vi "5_Creating_complex_analog_and_digital_sequences.vi"() -> ()   [LabVIEW 2014]
uses:
  <vilib>/Swabian Instruments/Pulse Streamer/PulseStreamer/PulseStreamer/typedefs/typedef_TriggerStart.ctl
  <vilib>/Swabian Instruments/Pulse Streamer/PulseStreamer/PulsePattern/PulsePattern.lvclass
  <vilib>/Swabian Instruments/Pulse Streamer/PulseStreamer/AnalogPattern/AnalogPattern.lvclass
  <vilib>/Swabian Instruments/Pulse Streamer/PulseStreamer/typedefs/typedef_ChannelNumber.ctl
  <vilib>/Swabian Instruments/Pulse Streamer/PulseStreamer/typedefs/typedef_OutputState.ctl
  <vilib>/Swabian Instruments/Pulse Streamer/PulseStreamer/Sequence/Sequence.lvclass/Sequence.ctl
  <vilib>/Swabian Instruments/Pulse Streamer/PulseStreamer/Pattern/Read total duration.vi
  <vilib>/Swabian Instruments/Pulse Streamer/PulseStreamer/PulseStreamer/stream/stream (Sequence).vi
  <vilib>/Swabian Instruments/Pulse Streamer/PulseStreamer/PulseStreamer/PulseStreamer.lvclass
  <vilib>/Swabian Instruments/Pulse Streamer/PulseStreamer/Sequence/Sequence.lvclass
  <vilib>/Swabian Instruments/Pulse Streamer/PulseStreamer/PulseStreamer.lvlib
panel:
  in  "ip":string="pulsestreamer"
  out "Total Duration [ns]":i64
  in  "Digital Pattern\nDuration [ns] & Level":cluster{"Duration [ns]":u64, "State":bool}[](array[cluster])=[{"Duration [ns]"=1000, "State"=FALSE}, {"Duration [ns]"=500, "State"=TRUE}, {"Duration [ns]"=200, "State"=FALSE}, {"Duration [ns]"=300, "State"=TRUE}, {"Duration [ns]"=100, "State"=FALSE}]
  in  "Level 3":bool
  in  "Duration 3":i64=250
  out "error out":errorcluster
  in  "nRuns":i64=1000
  in  "Start Trigger":T1
  in  "Repeat sequence":u32=5
  in  "Voltage A ch0-2":dbl min=-1.0 max=1.0
  in  "Voltage A ch0-1":dbl=1.0 min=-1.0 max=1.0
  in  "Duration A ch0-2":i64
  in  "Duration A ch0-1":i64=100
  in  "Duration 2":i64=500
  in  "Duration 1":i64=1000
  in  "Level 2":bool=TRUE
  in  "Level 1":bool
  # "This example demonstrates how to program each channel individually and how to combine them into sequence. \nThe durations of each pulse are automatically split so that the Generated sequence has the Run Length Encoding (RLE).\nThe total duration of a sequence has the length of the longest duration of all channels. \nThis example also shows few powerful techniques on how prepared sequences can be combined and repeated."
  # "INPUT SECTION"
  # "RESULT SECTION"
  # "Level 1"
  # "Level 2"
  # "Level 3"
  # "Duration"
  # "The longest duration is from channel 'Digital 0' and hence,\n this channel determines the total duration."
  # "either add single pulses"
  # "Digital 0"
  # "or a array of cluster\ntop: duration\nbutton: state [1: high, 0: low]"
  # "Digital 1"
  # "Level 1"
  # "Level 2"
  # "The very same is possible for the analog channels. Here only the method to add single pulses is shown.\nRemark:\nAdding a Pulse of duration 0 might be useful because this state will be padded until the maximum duration of all channels is reached."
  # "Duration"
  # "Analog 0"
  # "Sequence class has a repeat method which duplicates sequence data."
  # "StartTrigger: IMMEDIATE - starts streaming immediately after data received\nSOFTWARE - use \"startNow.vi\" as software trigger\nHW_RAISING, HW_FALLING, HW_RISING_AND_FALLING - tell Pulse Streamer to trigger by signal connected to \"Trigger\" input"
  # "If there is only one sequence 'nRuns' from the 'stream' method should\nbe always used, because with 'Repeat' the data transferred to the \nPulsestreamer is repeated 'Repeat' times whereas nRuns sends the sequence\nonly once.\nRepeat >1 should be used when several sequences are combined and \neach sequence needs to be repeated."
  # "Here you can define the state to set after the sequence\n streaming has finished."
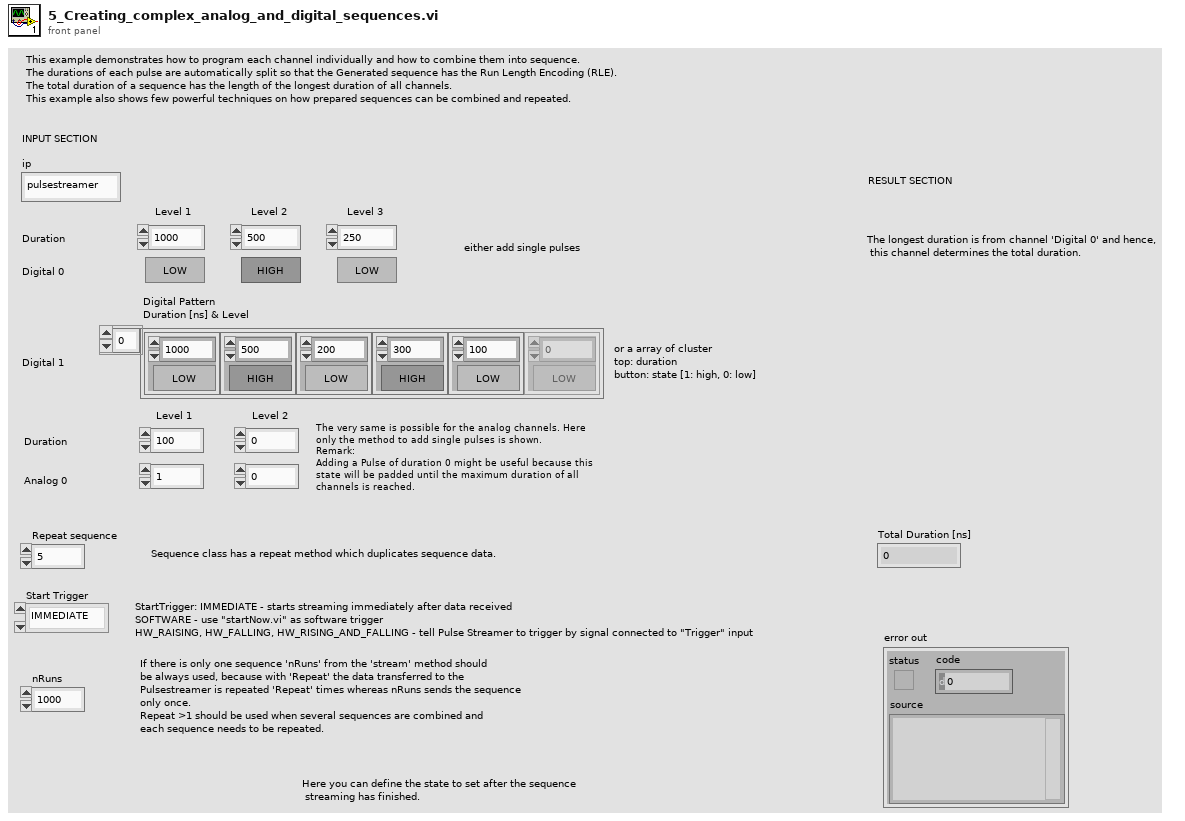
[diagram p1: front panel]
types:
  T1 = typedef "PulseStreamer.lvlib/PulseStreamer.lvclass/typedef_TriggerStart.ctl" = enum16{"IMMEDIATE", "SOFTWARE", "HW_RISING", "HW_FALLING", "HW_RISING_AND_FALLING"}
  T2 = typedef "PulseStreamer.lvlib/typedef_OutputState.ctl" = cluster{"channels":T3[], "a0":dbl, "a1":dbl}
  T3 = typedef "PulseStreamer.lvlib/typedef_ChannelNumber.ctl" = i16
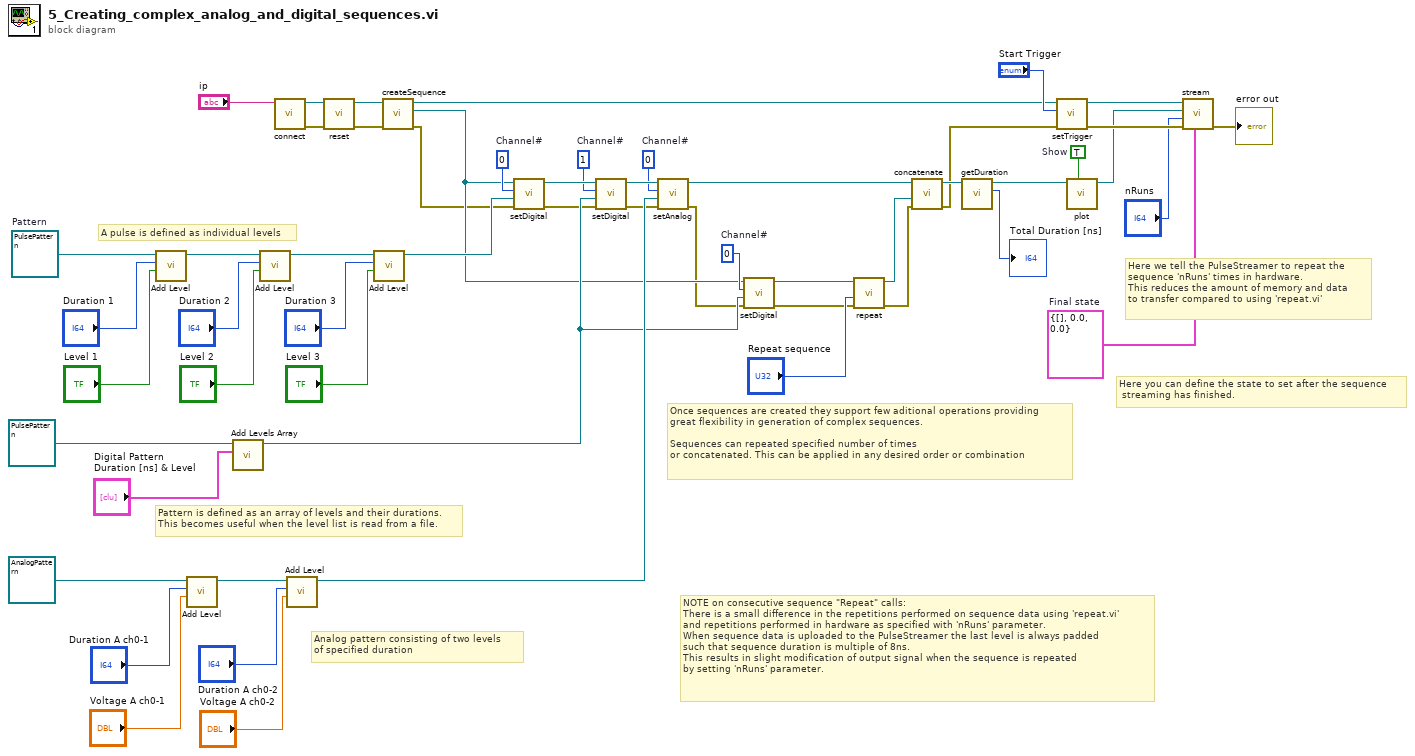
[diagram p0: block diagram]
diagram:
  w21 = T2 {"channels"=[], "a0"=0.0, "a1"=0.0}  # Final state
  w14 = TRUE  # Show
  w27 = T3 0  # Channel#
  w29 = T3 0  # Channel#
  w30 = T3 1  # Channel#
  w32 = T3 0  # Channel#
  w48 = refnum<class "PulsePattern.lvclass"> refnum  # Pattern
  # "Here you can define the state to set after the sequence\n streaming has finished."
  # "A pulse is defined as individual levels"
  # "NOTE on consecutive sequence \"Repeat\" calls: \nThere is a small difference in the repetitions performed on sequence data using 'repeat.vi'\nand repetitions performed in hardware as specified with 'nRuns' parameter.\nWhen sequence data is uploaded to the PulseStreamer the last level is always padded \nsuch that sequence duration is multiple of 8ns. \nThis results in slight modification of output signal when the sequence is repeated \nby setting 'nRuns' parameter."
  # "Here we tell the PulseStreamer to repeat the \nsequence 'nRuns' times in hardware.\nThis reduces the amount of memory and data\nto transfer compared to using 'repeat.vi'"
  # "Analog pattern consisting of two levels \nof specified duration"
  # "Pattern is defined as an array of levels and their durations.\nThis becomes useful when the level list is read from a file."
  # "Once sequences are created they support few aditional operations providing\ngreat flexibility in generation of complex sequences.\n\nSequences can repeated specified number of times \nor concatenated. This can be applied in any desired order or combination"
  n1 = call <vilib>:"Add Level.vi"("Level"="Level 1", "Duration"="Duration 1", "Digital Sequence in"=w48) -> ("Digital Sequence out"=w55:refnum<class "PulsePattern.lvclass">)  [unwired: 8 in]
  n2 = call <vilib>:"Add Level.vi"("Voltage"="Voltage A ch0-1", "Duration"="Duration A ch0-1", "Analog Sequence in"=refnum<class "AnalogPattern.lvclass"> refnum ("Analog Sequence.lvclass")) -> ("Analog Sequence out"=w53:refnum<class "AnalogPattern.lvclass">)  [unwired: 8 in]
  n3 = call-dynamic "Add Levels Array.vi"("Array of (Duration [ns], Level [T/F])"="Digital Pattern\nDuration [ns] & Level", "Digital Sequence in"=refnum<class "PulsePattern.lvclass"> refnum ("Digital Sequence.lvclass")) -> ("Digital Sequence out"=w25:refnum<class "PulsePattern.lvclass">)  [unwired: 9 in]
  n4 = call <vilib>:"Add Level.vi"("Level"="Level 2", "Duration"="Duration 2", "Digital Sequence in"=w55) -> ("Digital Sequence out"=w49:refnum<class "PulsePattern.lvclass">)  [unwired: 8 in]
  n5 = call <vilib>:"connect.vi"("ip"="ip") -> ("error out"=w23:errorcluster, "Pulse Streamer out"=w24:refnum<class "PulseStreamer.lvclass">)  [unwired: 9 in]
  n6 = call <vilib>:"Add Level.vi"("Voltage"="Voltage A ch0-2", "Duration"="Duration A ch0-2", "Analog Sequence in"=w53) -> ("Analog Sequence out"=w26:refnum<class "AnalogPattern.lvclass">)  [unwired: 8 in]
  n7 = call <vilib>:"reset.vi"("error in (no error)"=w23, "Pulse Streamer in"=w24) -> ("error out"=w9:errorcluster, "Pulse Streamer out"=w11:refnum<class "PulseStreamer.lvclass">)  [unwired: 8 in]
  n8 = call <vilib>:"Add Level.vi"("Level"="Level 3", "Duration"="Duration 3", "Digital Sequence in"=w49) -> ("Digital Sequence out"=w31:refnum<class "PulsePattern.lvclass">)  [unwired: 8 in]
  n9 = call-dynamic "createSequence.vi"("error in (no error)"=w9, "PulseStreamer in"=w11) -> ("error out"=w7:errorcluster, "Sequence"=w8:refnum<class "Sequence.lvclass">, "PulseStreamer out"=w10:refnum<class "PulseStreamer.lvclass">)  [unwired: 7 in]
  n10 = call-dynamic "setDigital.vi"("error in (no error)"=w7, "PulsePattern"=w31, "channel"=w32, "Sequence in"=w8) -> ("error out"=w6:errorcluster, "Sequence out"=w46:refnum<class "Sequence.lvclass">)  [unwired: 6 in]
  n11 = call-dynamic "setDigital.vi"("error in (no error)"=w6, "PulsePattern"=w25, "channel"=w30, "Sequence in"=w46) -> ("error out"=w5:errorcluster, "Sequence out"=w47:refnum<class "Sequence.lvclass">)  [unwired: 6 in]
  n12 = call-dynamic "setAnalog.vi"("error in (no error)"=w5, "AnalogPattern"=w26, "channel"=w29, "Sequence in"=w47) -> ("error out"=w4:errorcluster, "Sequence out"=w45:refnum<class "Sequence.lvclass">)  [unwired: 6 in]
  n13 = call-dynamic "setDigital.vi"("error in (no error)"=w4, "PulsePattern"=w25, "channel"=w27, "Sequence in"=w8) -> ("error out"=w3:errorcluster, "Sequence out"=w42:refnum<class "Sequence.lvclass">)  [unwired: 6 in]
  n14 = call <vilib>:"repeat.vi"("error in (no error)"=w3, "Repeat count"="Repeat sequence", "Sequence in"=w42) -> ("error out"=w2:errorcluster, "Sequence out"=w44:refnum<class "Sequence.lvclass">)  [unwired: 7 in]
  n15 = call <vilib>:"concatenate.vi"("error in (no error)"=w2, "Sequence to append"=w44, "Sequence in"=w45) -> ("error out"=w1:errorcluster, "Sequence out"=w41:refnum<class "Sequence.lvclass">)  [unwired: 7 in]
  n16 = call <vilib>:"getDuration.vi"("Sequence in"=w41) -> ("Sequence duration [ns]"=→"Total Duration [ns]":i64, "Sequence out"=w13:refnum<class "Sequence.lvclass">)  [unwired: 9 in]
  n17 = call-dynamic "setTrigger.vi"("error in (no error)"=w1, "start"="Start Trigger", "Pulse Streamer in"=w10) -> ("error out"=w39:errorcluster, "Pulse Streamer out"=w40:refnum<class "PulseStreamer.lvclass">)  [unwired: 7 in]
  n18 = call <vilib>:"plot.vi"("Show on call"=w14, "Sequence in"=w13) -> ("Sequence out"=w12:refnum<class "Sequence.lvclass">)  [unwired: 6 in, 3 out]
  n19 = call-poly <vilib>:"stream.vi"("final"=w21, "error in (no error)"=w39, "n_runs"="nRuns", "sequence"=w12, "Pulse Streamer in"=w40) -> ("error out"=→"error out":errorcluster)  [unwired: 3 in, 1 out]
